vi "TC Calibration Config.vi"(8 "error in (no error)":errorcluster, 11 "Node Ptr":T1 format="%.0x") -> (0 "error out":errorcluster)   [LabVIEW 2011, in "Simulated Thermocouple Custom Device.lvlib"]
uses:
  Simulated Thermocouple Custom Device.lvlib
  <vilib>/NI Veristand/Custom Device API/Custom Device Item Ref.ctl
  Calibration Config Data.ctl
  TC Selector.ctl
  <vilib>/NI Veristand/Custom Device API/Get Item Property (Variant).vi
  simTC Global GUIDs.vi
  <vilib>/NI Veristand/Custom Device Tools/Custom Device Utility Library/NI VeriStand - Search for All Items by GUID.vi
  <vilib>/NI Veristand/Custom Device API/Get Item Property (String).vi
  <vilib>/NI Veristand/Custom Device API/Set Item Property (Variant).vi
  <vilib>/regexp/Match Regular Expression.xnode
  <vilib>/NI Veristand/Custom Device API/Custom Device API.lvlib
  <vilib>/NI Veristand/Custom Device Tools/Custom Device Utility Library/Custom Device Utility Library.lvlib
panel:
  in  "Calibration Step Settling Time (s)":dbl=1.0
  in  "Calibration samples to collect":dbl=25.0
  in  "Local simTC Channel Output to calibrate on":u16(ring)
  in  "Header":cluster{"Section Name":string}={"Section Name"="Calibration Settings"}
  in  "Description":string="A calibration will require two channels:\n\n1.) A Simulated Thermocouple output from this custom device (Use selector below)\n2.) An external thermocouple input mapped to this channel in the system explorer\n\nThese channels must be physically connected via wires externally.  The measured value on this calibration channel will be compared to the desired output on the simulated thermocouple (select channel below) to determine error and calibration constants.\n\nTo perform the calibration, you must also select the number of points to sample.  20-30 points is tyically sufficient, although more may be needed if you plan to use the thermocouple near the upper or lower limits of its range."
  in  "Name":string
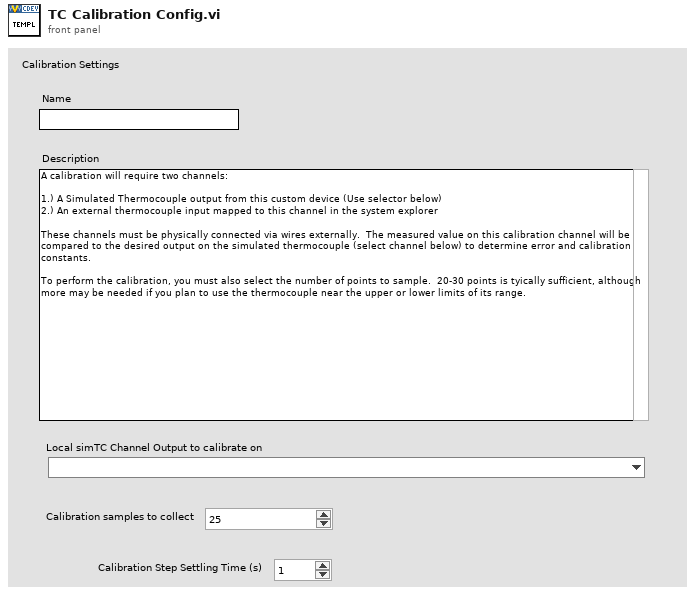
[diagram p1: front panel]
types:
  T1 = typedef "Custom Device API.lvlib/Custom Device Item Ref.ctl" = u64
  T2 = typedef "Simulated Thermocouple Custom Device.lvlib/Calibration Config Data.ctl" = cluster{"Local SimTC Chan":string, "Samples To Collect":dbl, "Cal Channel TC Type":T3, "Cal Step Settling Time":dbl}
  T3 = typedef "Simulated Thermocouple Custom Device.lvlib/TC Selector.ctl" = u16
  T4 = typedef "Custom Device API.lvlib/Custom Device Item Info.ctl" = cluster{"Name":string, "Is Channel":bool, "GUID":string}
  T5 = typedef "Custom Device API.lvlib/Custom Device Commands.ctl" = enum16{"Default", "Item renamed", "Shutdown", "Dynamic button pressed"}
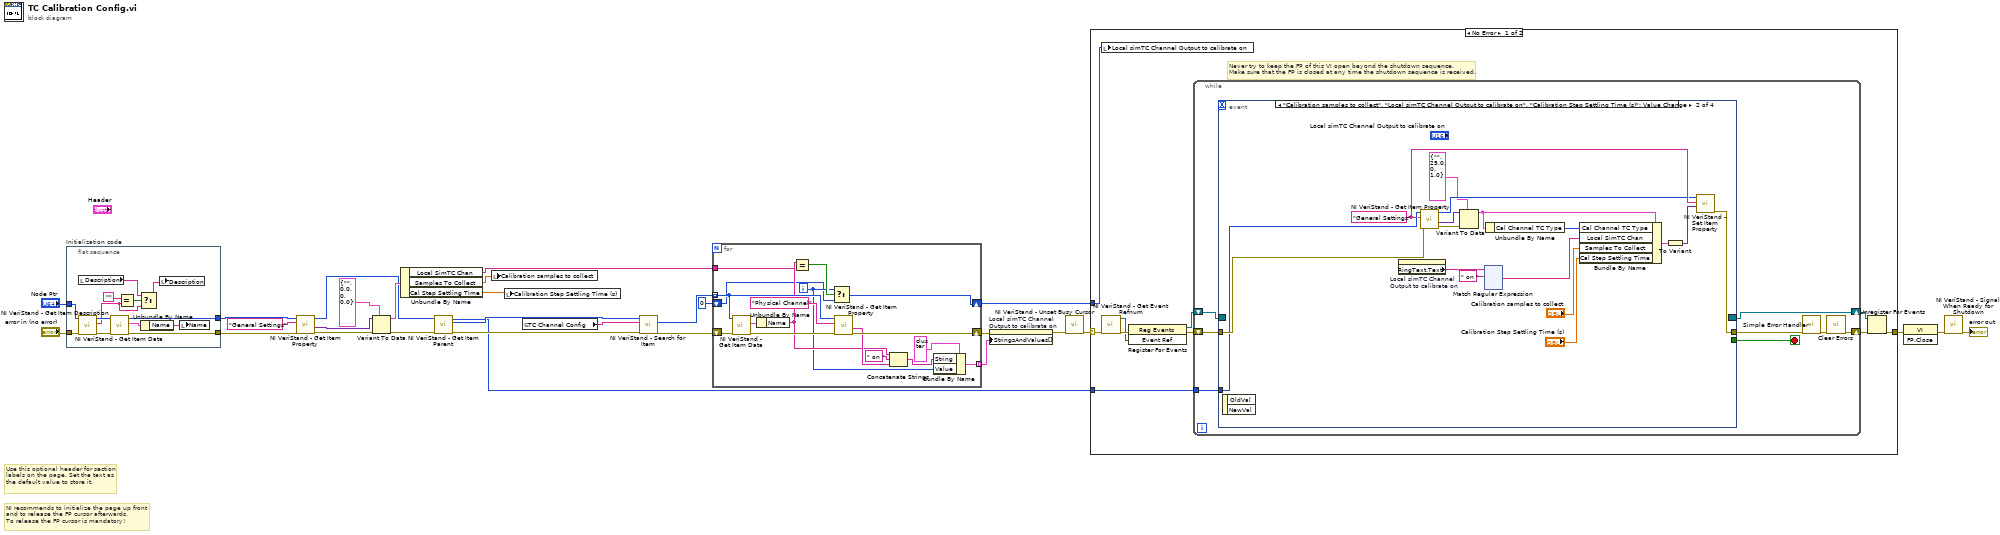
[diagram p0: block diagram]
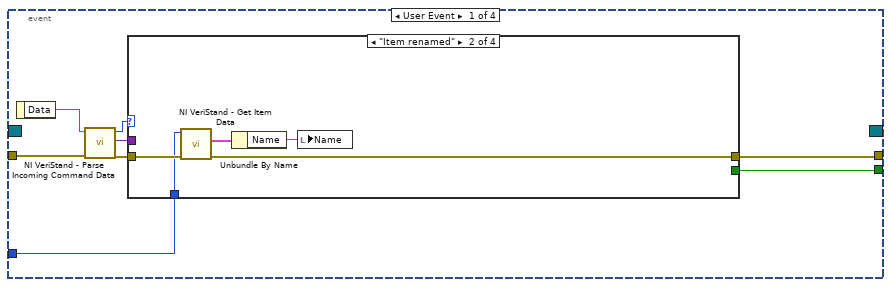
[diagram p2: hidden frame]
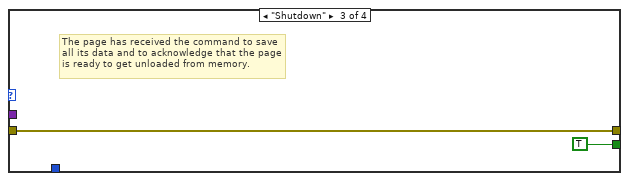
[diagram p4: hidden frame]
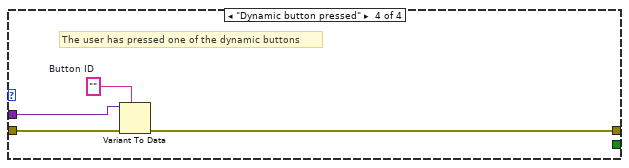
[diagram p5: hidden frame]
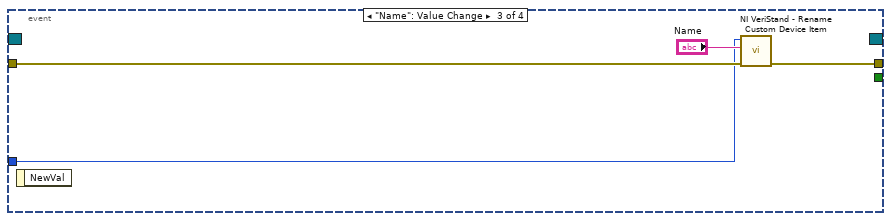
[diagram p6: hidden frame]
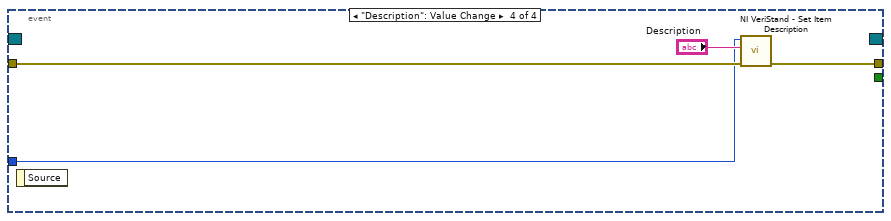
[diagram p7: hidden frame]
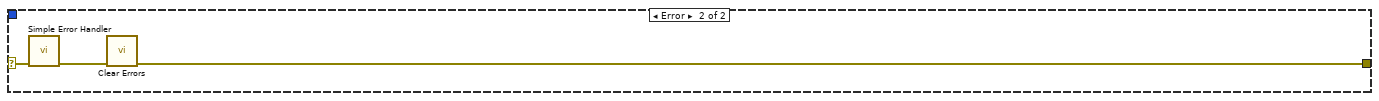
[diagram p8: hidden frame]
diagram:
  # "Use this optional header for section labels on the page. Set the text as the default value to store it."
  # "NI recommends to initialize the page up front\nand to release the FP cursor afterwards.\nTo release the FP cursor is mandatory!"
  n1 = flat-sequence "Initialization code" {
    tunnel: "error in (no error)" -> [w40]
    tunnel: "Node Ptr" -> [w39]
    tunnel: [w35] -> w16
    tunnel: [w42] -> w17
    frame #0 {
      n2 = call <vilib>:"NI VeriStand - Get Item Description.vi"("error in (no error)"=w40, "Item Ref in"=w39) -> ("error out"=w38:errorcluster, "Description"=w30:string, "Item Ref out"=w41:T1)  [unwired: 7 out]
      n3 = local read "Description"() -> (w32:string)
      n4 = call <vilib>:"NI VeriStand - Get Item Data.vi"("error in (no error)"=w38, "Item Ref in"=w41) -> ("error out"=w35:errorcluster, "Item Info"=w37:T4, "Item Ref out"=w42:T1)  [unwired: 7 out]
      n5 = Equal?(x="", y=w30) -> (x = y?=w34:bool)
      n6 = Select(t=w32, s=w34, f=w30) -> (s? t:f=w31:string)
      n7 = Unbundle By Name(w37) -> ("Name"=w36:string)
      n8 = local write "Description"(w31) -> ()
      n9 = local write "Name"(w36) -> ()
    }
  }
  n10 = call-poly <vilib>:"NI VeriStand - Get Item Property.vi"("error in (no error)"=w16, "Property Name"="General Settings", "Item Ref in"=w17) -> ("error out"=w14:errorcluster, "Value"=w13:variant, "Item Ref out"=w3:T1)  [unwired: 5 in, 1 out]
  n11 = Variant To Data(error in=w14, type=T2 {"Local SimTC Chan"="", "Samples To Collect"=0.0, "Cal Channel TC Type"=0, "Cal Step Settling Time"=0.0} ("Cal Info"), Variant=w13) -> (data=w10:T2, error out=w11:errorcluster)
  n12 = Unbundle By Name(w10) -> ("Local SimTC Chan"=w9:string, "Samples To Collect"=w4:dbl, "Cal Step Settling Time"=w1:dbl)
  n13 = call <vilib>:"NI VeriStand - Get Item Parent.vi"("error in (no error)"=w11, "Item Ref in"=w3) -> ("error out"=w22:errorcluster, "Parent Ref"=w21:T1, "Item Ref out"=w2:T1)  [unwired: 6 in, 1 out]
  n14 = local write "Calibration samples to collect"(w4) -> ()
  n15 = local write "Calibration Step Settling Time (s)"(w1) -> ()
  n16 = global read "simTC Global GUIDs.vi" "TC Channel Config"() -> (w23:string)
  n17 = call-poly <vilib>:"NI VeriStand - Search for Item.vi"("error in"=w22, "Item GUID"=w23, "Section Ref in"=w21) -> ("error out"=w19:errorcluster, "Item Refs"=w20:T1[])  [unwired: 5 in, 2 out]
  n18 = for {
    tunnel: w20 -> [w58] mode=indexing
    tunnel: [w49] -> w18 mode=indexing
    shift-right: [w54] -> w5
    shift-left: w19 -> [w56]
    tunnel: w9 -> [w47]
    shift-right: [w46] -> w7
    shift-left: 0 -> [w43]
    i -> [w44]
    n19 = call <vilib>:"NI VeriStand - Get Item Data.vi"("error in (no error)"=w56, "Item Ref in"=w58) -> ("error out"=w55:errorcluster, "Item Info"=w59:T4)  [unwired: 8 out]
    n20 = Unbundle By Name(w59) -> ("Name"=w48:string)
    n21 = Equal?(x=w48, y=w47) -> (x = y?=w45:bool)
    n22 = Select(t=w44, s=w45, f=w43) -> (s? t:f=w46:i32)
    n23 = call-poly <vilib>:"NI VeriStand - Get Item Property.vi"("error in (no error)"=w55, "Property Name"="Physical Channel", "Item Ref in"=w58) -> ("error out"=w54:errorcluster, "Value"=w52:string)  [unwired: 5 in, 2 out]
    n24 = Concatenate Strings(w48, " on " ("string"), w52) -> (w51:string)
    n25 = Bundle By Name(cluster=cluster{"String":string, "Value":ext} {"String"="", "Value"=0.0}, "String"=w51, "Value"=w44) -> (w49:cluster{"String":string, "Value":ext})
  }
  n26 = property on="Local simTC Channel Output to calibrate on" class="Ring (strict)"(error in=w5, "StringsAndValues[]"=w18) -> (error out=w6:errorcluster)  [unwired: 1 in, 1 out]
  n27 = call <vilib>:"NI VeriStand - Unset Busy Cursor.vi"("error in (no error)"=w6) -> ("error out"=w25:errorcluster)  [unwired: 10 out]
  n28 = case shown="No Error" w25 {
    selector: w25 -> [w62 w236]
    tunnel: [w66 w234] -> w29
    tunnel: w7 -> [w61 _]
    tunnel: w2 -> [w60 _]
    frame No Error {
      # "Never try to keep the FP of this VI open beyond the shutdown sequence.\nMake sure that the FP is closed at any time the shutdown sequence is received."
      n29 = local write "Local simTC Channel Output to calibrate on"(w61) -> ()
      n30 = call <vilib>:"NI VeriStand - Get Event Refnum.vi"("error in (no error)"=w62) -> ("error out"=w69:errorcluster, "Event Ref"=w65:refnum<user-event>)  [unwired: 9 out]
      n31 = register-events(error in=w69, w65) -> (reference out=w63:refnum<event-registration>, error out=w64:errorcluster)  [unwired: 1 in]
      n32 = while {
        shift-right: [w71] -> w67
        shift-left: w64 -> [w76]
        shift-right: [w77] -> w68
        shift-left: w63 -> [w75]
        tunnel: w60 -> [w70]
        stop <- w74 stop-if-true
        n33 = event shown="[1] \"Calibration samples to collect\", \"Local simTC Channel Output to calibrate on\", \"Calibration Step Settling Time (s)\": Value Change" {
          selector: w75 -> [_ _ _ _]
          dyn-events: [_ _ _ _] -> w77
          timeout: _ -> [_ _ _ _]
          tunnel: w76 -> [w85 w107 w229 w233]
          tunnel: [w81 _ _ _] -> w74
          tunnel: [w80 w109 w228 w232] -> w73
          tunnel: w70 -> [w78 w104 w226 w230]
          event User Event {
            n34 = event-data() -> ("Data"=w84:string)  [unwired: 1 out]
            n35 = call <vilib>:"NI VeriStand - Parse Incoming Command Data.vi"("error in (no error)"=w85, "Incoming data"=w84) -> ("error out"=w83:errorcluster, "Outgoing data"=w79:variant, "Action"=w82:T5)  [unwired: 7 out]
            n36 = case shown="\"Item renamed\"" w82 {
              tunnel: w83 -> [w86 w91 w92 w97]
              tunnel: [_ _ TRUE _] -> w81
              tunnel: [w86 w89 w92 w94] -> w80
              tunnel: w79 -> [_ _ _ w96]
              tunnel: w78 -> [_ w87 _ _]
              frame "Default", Default {
              }
              frame "Item renamed" {
                n37 = call <vilib>:"NI VeriStand - Get Item Data.vi"("error in (no error)"=w91, "Item Ref in"=w87) -> ("error out"=w89:errorcluster, "Item Info"=w90:T4)  [unwired: 8 out]
                n38 = Unbundle By Name(w90) -> ("Name"=w88:string)
                n39 = local write "Name"(w88) -> ()
              }
              frame "Shutdown" {
                # "The page has received the command to save all its data and to acknowledge that the page is ready to get unloaded from memory."
              }
              frame "Dynamic button pressed" {
                w95 = ""  # Button ID
                # "The user has pressed one of the dynamic buttons"
                n40 = Variant To Data(error in=w97, type=w95, Variant=w96) -> (error out=w94:errorcluster)  [unwired: 1 out]
              }
            }
          }
          event "Calibration samples to collect", "Local simTC Channel Output to calibrate on", "Calibration Step Settling Time (s)": Value Change {
            w103 = "General Settings" ("Property Name")
            n41 = event-data() -> ()  [unwired: 3 out]
            n42 = property on="Local simTC Channel Output to calibrate on" class="Ring (strict)"() -> ("RingText.Text"=w114:string)  [unwired: 2 in, 2 out]
            n43 = call-poly <vilib>:"NI VeriStand - Get Item Property.vi"("error in (no error)"=w107, "Property Name"=w103, "Item Ref in"=w104) -> ("error out"=w106:errorcluster, "Value"=w105:variant, "Item Ref out"=w102:T1)  [unwired: 5 in, 1 out]
            n44 = Variant To Data(error in=w106, type=T2 {"Local SimTC Chan"="", "Samples To Collect"=25.0, "Cal Channel TC Type"=0, "Cal Step Settling Time"=1.0} ("Cal Info"), Variant=w105) -> (data=w100:T2)  [unwired: 1 out]
            n45 = xnode "Match Regular Expression"("input string"=w114, "regular expression"=" on ") -> ("after match"=w98:string)  [unwired: 4 in, 4 out]
            n46 = Unbundle By Name(w100) -> ("Cal Channel TC Type"=w99:T3)
            n47 = Bundle By Name(cluster=w100, "Cal Channel TC Type"=w99, "Local SimTC Chan"=w98, "Samples To Collect"="Calibration samples to collect", "Cal Step Settling Time"="Calibration Step Settling Time (s)") -> (w111:T2)
            n48 = To Variant(anything=w111) -> (Variant=w110:variant)
            n49 = call-poly <vilib>:"NI VeriStand - Set Item Property.vi"("Value"=w110, "Property Name"=w103, "Item Ref in"=w102) -> ("error out"=w109:errorcluster)  [unwired: 6 in, 2 out]
          }
          event "Name": Value Change {
            n50 = event-data() -> ()  [unwired: 2 out]
            n51 = call <vilib>:"NI VeriStand - Rename Custom Device Item.vi"("error in (no error)"=w229, "New Name"="Name", "Item Ref in"=w226) -> ("error out"=w228:errorcluster)  [unwired: 8 out]
          }
          event "Description": Value Change {
            n52 = event-data() -> ()  [unwired: 2 out]
            n53 = call <vilib>:"NI VeriStand - Set Item Description.vi"("error in (no error)"=w233, "Description"="Description", "Item Ref in"=w230) -> ("error out"=w232:errorcluster)  [unwired: 8 out]
          }
        }
        n54 = call <vilib>:"Simple Error Handler.vi"("error in (no error)"=w73) -> ("error out"=w72:errorcluster)  [unwired: 1 in, 7 out]
        n55 = call <vilib>:"Clear Errors.vi"("error in (no error)"=w72) -> ("error out"=w71:errorcluster)  [unwired: 6 out]
      }
      n56 = Unregister For Events(event registration refnum=w68, error in=w67) -> (error out=w66:errorcluster)
    }
    frame Error {
      n57 = call <vilib>:"Simple Error Handler.vi"("error in (no error)"=w236) -> ("error out"=w235:errorcluster)  [unwired: 1 in, 7 out]
      n58 = call <vilib>:"Clear Errors.vi"("error in (no error)"=w235) -> ("error out"=w234:errorcluster)  [unwired: 6 out]
    }
  }
  n59 = invoke class="VI" method="FP.Close"(error in=w29) -> (error out=w28:errorcluster)  [unwired: 2 in, 2 out]
  n60 = call <vilib>:"NI VeriStand - Signal When Ready for Shutdown.vi"("error in (no error)"=w28) -> ("error out"=→"error out":errorcluster)  [unwired: 10 out]
